vi "reward_behavior_timeout_12s_probes.vi"() -> ()   [LabVIEW 2019]
doc: "The myRIO Project template acquires acceleration data from the onboard accelerometer and displays the changes of acceleration values in a waveform chart."
uses:
  <vilib>/Analysis/Matrix/Datatypes/RealMatrix.ctl
  <vilib>/myRIO/Common/Instrument Driver Framework/myRIO v1.0/Encoder/typedefs/Encoder Signal Mode.ctl
  <vilib>/myRIO/Instrument Drivers/Onboard IO/Encoder/typedefs/Encoder Reference.ctl
  <vilib>/myRIO/Common/Instrument Driver Framework/Utilities/typedefs/myRIO Generic Hardware Reference.ctl
  <vilib>/myRIO/Common/Instrument Driver Framework/Utilities/typedefs/Hardware Version Enum.ctl
  <vilib>/myRIO/Common/Instrument Driver Framework/Utilities/typedefs/myRIO v1.0 Reference.ctl
  <vilib>/myRIO/Common/Instrument Driver Framework/Utilities/typedefs/Generic FPGA Reference.ctl
  <vilib>/myRIO/Common/Instrument Driver Framework/myRIO v1.0/Encoder/typedefs/Encoder Channels Enum.ctl
  <vilib>/myRIO/Common/Instrument Driver Framework/myRIO v1.0/Encoder/typedefs/Encoder Configuration v1.0.ctl
  <vilib>/userdefined/High Color/nirio_resource_hc.ctl
  <vilib>/myRIO/Instrument Drivers/Onboard IO/DIO/typedefs/DIO Reference.ctl
  <vilib>/myRIO/Common/Instrument Driver Framework/myRIO v1.0/DIO/typedefs/DIO Channels List.ctl
  <vilib>/myRIO/Common/Instrument Driver Framework/myRIO v1.0/DIO/typedefs/DIO Channels Enum.ctl
  <vilib>/myRIO/Common/Instrument Driver Framework/Utilities/vis/Is FPGA Ref Available.vi
  <vilib>/myRIO/Common/Instrument Driver Framework/myRIO v1.0/Encoder/vis/myRIO v1.1 Open Encoder.vi
  <vilib>/myRIO/Instrument Drivers/Onboard IO/Encoder/vis/Read.vi
  <vilib>/myRIO/Common/Instrument Driver Framework/myRIO v1.0/DIO/vis/myRIO v1.1 Open DIO.vi
  <vilib>/myRIO/Instrument Drivers/Onboard IO/DIO/vis/Write.vi
  <vilib>/myRIO/Instrument Drivers/Onboard IO/DIO/vis/Read.vi
  <vilib>/myRIO/Common/Instrument Driver Framework/Utilities/vis/Validate Channels.vi
  <vilib>/myRIO/Common/Instrument Driver Framework/myRIO v1.0/Encoder/vis/myRIO v1.0 Reserve Encoder.vi
  <vilib>/myRIO/Common/Instrument Driver Framework/myRIO v1.0/DIO/vis/myRIO v1.0 Reserve DIO.vi
  <vilib>/myRIO/Common/Instrument Driver Framework/myRIO v1.0/Encoder/vis/myRIO v1.0 Build MUX Configuration Encoder.vi
  <vilib>/myRIO/Common/Instrument Driver Framework/myRIO v1.0/Resource Manager/vis/myRIO v1.0 Reserve Channel List.vi
  <vilib>/myRIO/Common/Instrument Driver Framework/myRIO v1.0/DIO/vis/myRIO v1.0 Build MUX Configuration DIO.vi
  <vilib>/myRIO/Common/Instrument Driver Framework/myRIO v1.0/Resource Manager/vis/myRIO v1.0 Create Configuration List.vi
  <vilib>/myRIO/Common/Instrument Driver Framework/myRIO v1.0/Resource Manager/vis/myRIO v1.0 Reserve Channel.vi
  <vilib>/myRIO/Common/Instrument Driver Framework/myRIO v1.0/Resource Manager/vis/myRIO v1.0 Unreserve Channel.vi
  <vilib>/myRIO/Common/Instrument Driver Framework/myRIO v1.0/Resource Manager/vis/myRIO v1.0 Build Mutex Name.vi
  <vilib>/Utility/VariantDataType/GetNumericInfo.vi
  <vilib>/Utility/error.llb/Error Cluster From Error Code.vi
  <vilib>/myRIO/Common/Instrument Driver Framework/myRIO v1.0/myRIO v1.1 Open.vi
  <vilib>/myRIO/Common/Instrument Driver Framework/Utilities/vis/IO Manager.vi
  <vilib>/myRIO/Common/Instrument Driver Framework/Utilities/vis/Configuration Manager.vi
  <vilib>/myRIO/Common/Instrument Driver Framework/myRIO v1.0/Resource Manager/vis/myRIO v1.0 Configure IO.vi
  <vilib>/myRIO/Common/Instrument Driver Framework/myRIO v1.0/myRIO v1.0 Close.vi
  <vilib>/myRIO/Common/Instrument Driver Framework/myRIO v1.0/Encoder/vis/myRIO v1.0 Configure Encoder.vi
  <vilib>/myRIO/Common/Instrument Driver Framework/myRIO v1.0/Encoder/vis/myRIO v1.0 Read Encoder.vi
  <vilib>/myRIO/Common/Instrument Driver Framework/myRIO v1.0/DIO/vis/myRIO v1.0 Read DIO.vi
  <vilib>/myRIO/Common/Instrument Driver Framework/myRIO v1.0/DIO/vis/myRIO v1.0 Write DIO.vi
  <vilib>/myRIO/Express VI/Onboard IO/Encoder/Encoder Express VI.xnode
  <vilib>/myRIO/Instrument Drivers/Onboard IO/Encoder/vis/myRIO Encoder Open.xnode
  <vilib>/myRIO/Express VI/Onboard IO/DI/DI Express VI.xnode
  <vilib>/myRIO/Instrument Drivers/Onboard IO/DIO/vis/myRIO DIO Open.xnode
  <vilib>/myRIO/Express VI/Onboard IO/DO/DO Express VI.xnode
  <vilib>/myRIO/Instrument Drivers/Onboard IO/Encoder/Encoder.lvlib
  <vilib>/myRIO/Instrument Drivers/Onboard IO/DIO/DIO.lvlib
  <vilib>/Analysis/Matrix/NI_Matrix.lvlib
panel:
  out "Timings":dbl[](array[numeric])
  out "ISI":dbl
  out "ISI start time":dbl
  out "Time_out":bool=TRUE
  out "Time since lick":dbl
  out "Time of last lick":dbl
  out "Rewarded trials":dbl[](array[numeric])
  out "Rewards":u16
  out "Active Trial":bool
  out "Array temp2":T1
  out "Stimuli Loaded":bool
  out "Stim_ID":dbl[](array[numeric])
  out "Reward_mat":dbl[](array[numeric])
  out "Reward":bool=TRUE
  out "Frame clock":i32
  out "Licks":u32
  out "Lick":bool
  out "Time":dbl
  out "Stop":bool
  in  "Frames to collect":u32
  out "Overflow?":bool
  out "Counter Value":i32
  out "Velocity":dbl
  out "Velocity Plot":dbl[](graph)
  out "Velocity array":dbl[](array[numeric])
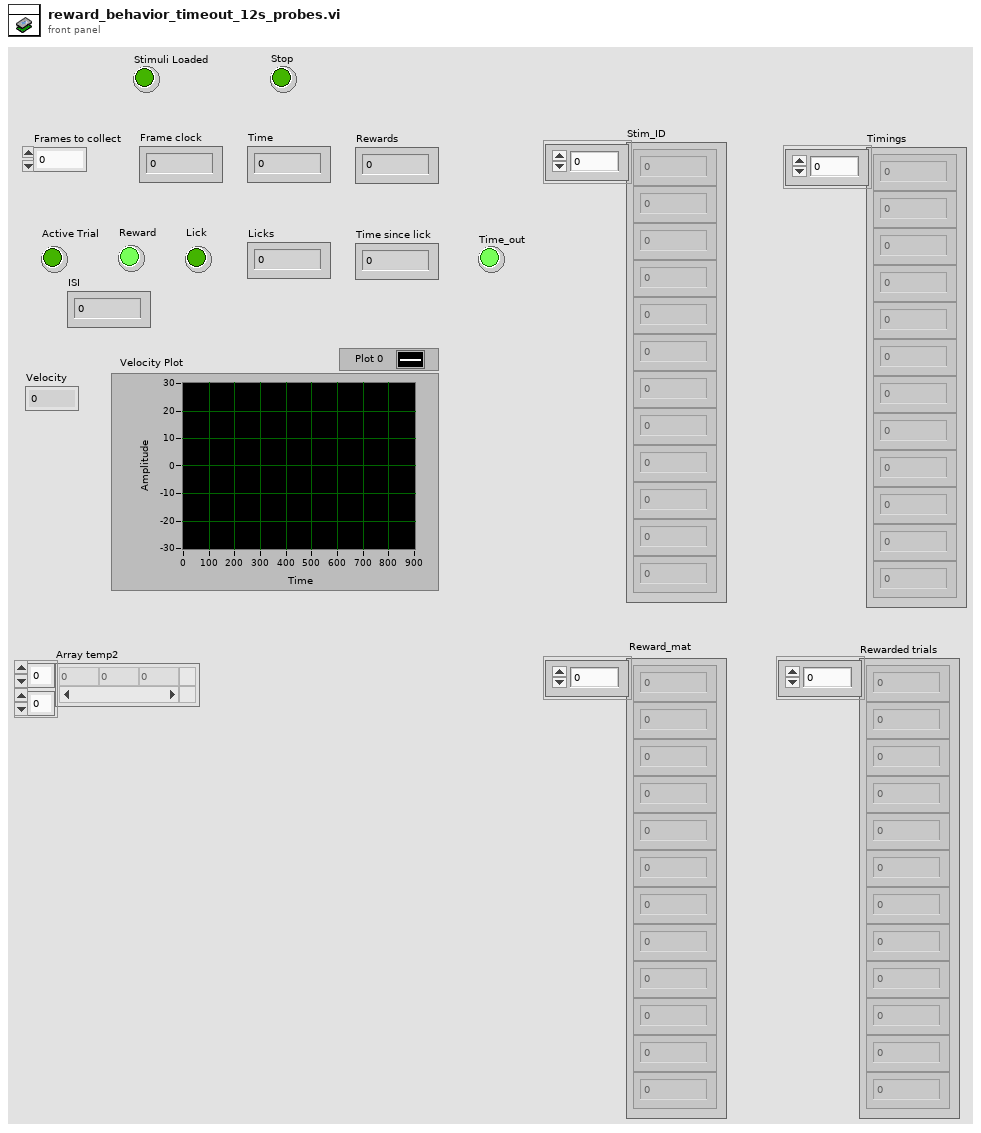
[diagram p1: front panel]
types:
  T1 = typedef "NI_Matrix.lvlib/RealMatrix.ctl" = dbl[][]
  T2 = typedef "Encoder.lvlib/Encoder Reference.ctl" = cluster{"myRIO Reference":T3, "Encoder Channels Enum":T7}
  T3 = typedef "myRIO Generic Hardware Reference.ctl" = cluster{"myRIO Model":T4, "myRIO Hardware Reference":T5}
  T4 = typedef "Hardware Version Enum.ctl" = enum16{"Unknown", "myRIO-1900", "myRIO-1950", "roboRIO", "NI ELVIS RIO CM", "ELVIS III"}
  T5 = typedef "myRIO v1.0 Reference.ctl" = cluster{"Generic FPGA Reference":T6, "Allow multiple opens":bool}
  T6 = typedef "Generic FPGA Reference.ctl" = refnum<k20>
  T7 = typedef "Encoder Channels Enum.ctl" = enum16{"Not Connected", "C/ENC0", "C/ENC1", "A/ENC", "A/ENC0", "A/ENC1", "A/ENC2", "A/ENC3", "A/ENC4", "A/ENC5", "A/ENC6", "A/ENC7", "A/ENC8", "A/ENC9", "B/ENC", "B/ENC0", "B/ENC1", "B/ENC2", "B/ENC3", "B/ENC4", "B/ENC5", "B/ENC6", "B/ENC7", "B/ENC8", "B/ENC9", "DIO/ENC0", "DIO/ENC1", "DIO/ENC2", "DIO/ENC3", "DIO/ENC4"}
  T8 = typedef "Encoder Signal Mode.ctl" = enum16{"Quadrature phase signal", "Step and direction signal"}
  T9 = typedef "nirio_resource_hc.ctl" = tag
  T10 = typedef "DIO.lvlib/DIO Reference.ctl" = cluster{"myRIO Reference":T3, "DIO Channels List":T11}
  T11 = typedef "DIO Channels List.ctl" = T12[]
  T12 = typedef "DIO Channels Enum.ctl" = enum16{"Not Connected", "C/DIO0", "C/DIO1", "C/DIO2", "C/DIO3", "C/DIO4", "C/DIO5", "C/DIO6", "C/DIO7", "A/DIO0", "A/DIO1", "A/DIO2", "A/DIO3", "A/DIO4", "A/DIO5", "A/DIO6", "A/DIO7", "A/DIO8", "A/DIO9", "A/DIO10", "A/DIO11", "A/DIO12", "A/DIO13", "A/DIO14", "A/DIO15", "A/DIO16", "A/DIO17", "A/DIO18", "A/DIO19", "B/DIO0", "B/DIO1", "B/DIO2", "B/DIO3", "B/DIO4", "B/DIO5", "B/DIO6", "B/DIO7", "B/DIO8", "B/DIO9", "B/DIO10", "B/DIO11", "B/DIO12", "B/DIO13", "B/DIO14", "B/DIO15", "B/DIO16", "B/DIO17", "B/DIO18", "B/DIO19", "LED0", "LED1", "LED2", "LED3", "Button0", "DIO/DIO0", "DIO/DIO1", "DIO/DIO2", "DIO/DIO3", "DIO/DIO4", "DIO/DIO5", "DIO/DIO6", "DIO/DIO7", "DIO/DIO8", "DIO/DIO9", "SPI/CS0", "SPI/CS1", "SPI/CS2", "SPI/CS3", "LED RADIO (Green)", "LED RADIO (Red)", "LED COMM (Green)", "LED COMM (Red)", "LED MODE (Green)", "LED MODE (Red)"}
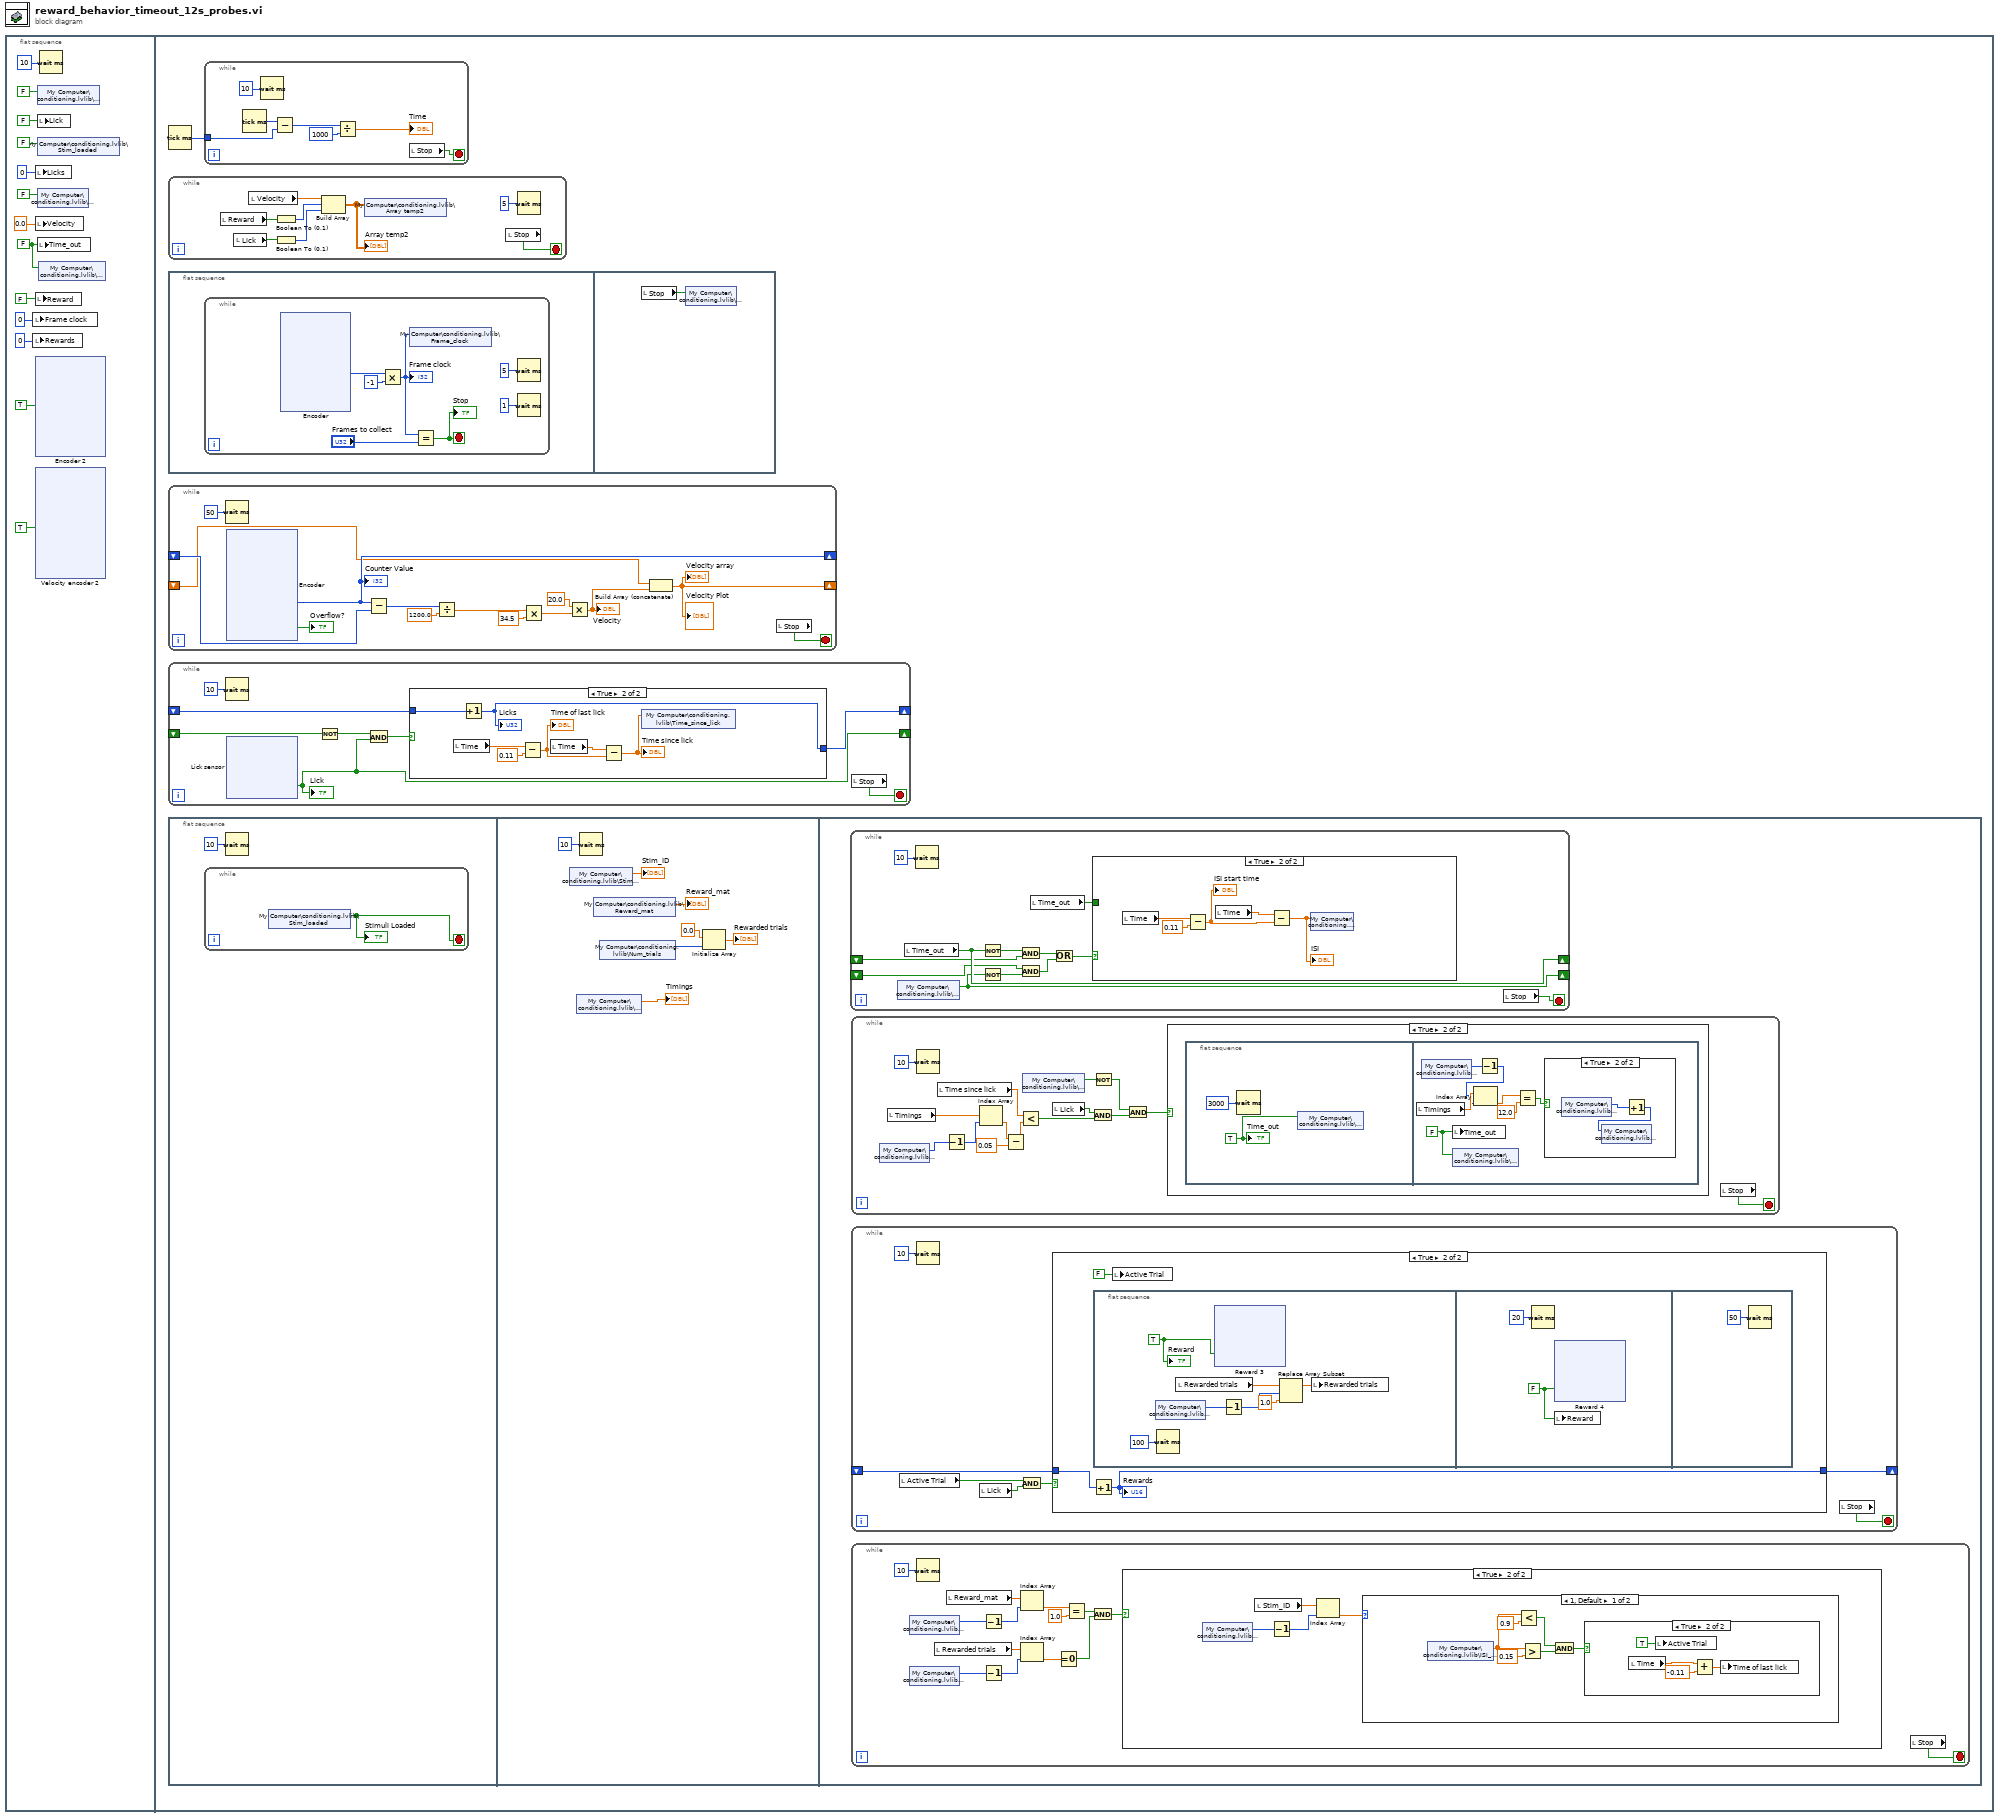
[diagram p0: block diagram]
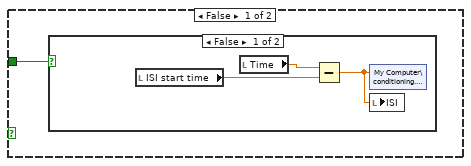
[diagram p4: hidden frame]
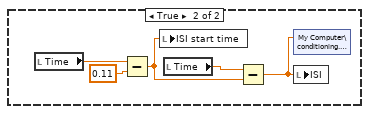
[diagram p5: hidden frame]
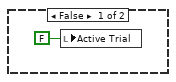
[diagram p6: hidden frame]
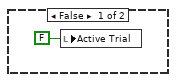
[diagram p7: hidden frame]
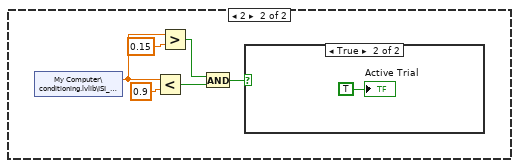
[diagram p8: hidden frame]
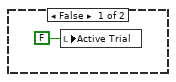
[diagram p9: hidden frame]
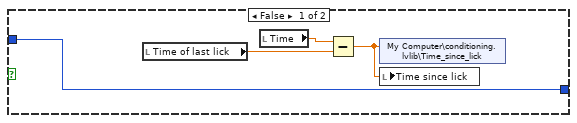
[diagram p11: hidden frame]
diagram:
  n1 = flat-sequence {
    frame #0 {
      w1 = FALSE ("Time_out")
      n2 = local write "Frame clock"(u32 0 ("Frames")) -> ()
      n3 = local write "Rewards"(u16 0 ("Rewards")) -> ()
      n4 = local write "Licks"(u32 0 ("Licks")) -> ()
      n5 = local write "Velocity"(0.0 ("Velocity")) -> ()
      n6 = local write "Reward"(FALSE ("Give reward")) -> ()
      n7 = xnode "Encoder 2"("Reset Counter"=TRUE) -> ()  [unwired: 1 in, 4 out]
      n8 = xnode "Velocity encoder 2"("Reset Counter"=TRUE) -> ()  [unwired: 1 in, 4 out]
      n9 = shared-variable "My Computer\\conditioning.lvlib\\Display"(FALSE ("Display")) -> ()  [unwired: 1 in, 1 out]
      n10 = local write "Lick"(FALSE ("Lick")) -> ()
      n11 = shared-variable "My Computer\\conditioning.lvlib\\Stim_loaded"(FALSE ("Stim_loaded")) -> ()  [unwired: 1 in, 1 out]
      n12 = shared-variable "My Computer\\conditioning.lvlib\\Stop"(FALSE ("Stop")) -> ()  [unwired: 1 in, 1 out]
      n13 = local write "Time_out"(w1) -> ()
      n14 = shared-variable "My Computer\\conditioning.lvlib\\Timeout"(w1) -> ()  [unwired: 1 in, 1 out]
      n15 = Wait (ms)(milliseconds to wait=u32 10) -> ()  [unwired: 1 out]
    }
    frame #1 {
      n16 = Tick Count (ms)() -> (millisecond timer value=w106:u32)
      n17 = while {
        stop <- w108 stop-if-true
        n18 = local read "Reward"() -> (w113:bool)
        n19 = local read "Lick"() -> (w114:bool)
        n20 = local read "Velocity"() -> (w112:dbl)
        n21 = Boolean To (0,1)(Boolean=w113) -> (0, 1=w111:i16)
        n22 = Boolean To (0,1)(Boolean=w114) -> (0, 1=w110:i16)
        n23 = Build Array(w112, w111, w110) -> (w107:T1)
        "Array temp2" <- w107
        n24 = shared-variable "My Computer\\conditioning.lvlib\\Array temp2"(w107) -> ()  [unwired: 1 in, 1 out]
        n25 = local read "Stop"() -> (w108:bool)
        n26 = Wait (ms)(milliseconds to wait=u32 5) -> ()  [unwired: 1 out]
      }
      n27 = flat-sequence {
        frame #0 {
          n28 = while {
            stop <- w306 stop-if-true
            n29 = xnode "Encoder"() -> ("Counter Value"=w310:i32)  [unwired: 2 in, 3 out]
            n30 = Multiply(x=w310, y=-1) -> (x*y=w305:i32)
            "Frame clock" <- w305
            n31 = shared-variable "My Computer\\conditioning.lvlib\\Frame_clock"(w305) -> ()  [unwired: 1 in, 1 out]
            n32 = Equal?(x=w305, y="Frames to collect") -> (x = y?=w306:bool)
            "Stop" <- w306
            n33 = Wait (ms)(milliseconds to wait=u32 5) -> ()  [unwired: 1 out]
            n34 = Wait (ms)(milliseconds to wait=u32 1) -> ()  [unwired: 1 out]
          }
        }
        frame #1 {
          n35 = local read "Stop"() -> (w358:bool)
          n36 = shared-variable "My Computer\\conditioning.lvlib\\Stop"(w358) -> ()  [unwired: 1 in, 1 out]
        }
      }
      n37 = while {
        shift-right: [w423] -> _
        shift-left: _ -> [w424]
        shift-right: [w415] -> _
        shift-left: _ -> [w414]
        stop <- w413 stop-if-true
        n38 = Wait (ms)(milliseconds to wait=u32 50) -> ()  [unwired: 1 out]
        n39 = xnode "Encoder"() -> ("Counter Value"=w423:i32, "Overflow?"=→"Overflow?":bool)  [unwired: 2 in, 2 out]
        "Counter Value" <- w423
        n40 = Subtract(x=w423, y=w424) -> (x-y=w416:i32)
        n41 = Divide(x=w416, y=1200.0 ("600")) -> (x/y=w421:dbl)
        n42 = Multiply(x=w421, y=34.5) -> (x*y=w419:dbl)
        n43 = Multiply(x=20.0, y=w419) -> (x*y=w417:dbl)
        "Velocity" <- w417
        n44 = Build Array (concatenate)(w414, w417) -> (w415:dbl[])
        "Velocity Plot" <- w415
        "Velocity array" <- w415
        n45 = local read "Stop"() -> (w413:bool)
      }
      n46 = while {
        shift-right: [w365] -> _
        shift-left: _ -> [w364]
        shift-right: [w359] -> _
        shift-left: _ -> [w362]
        stop <- w363 stop-if-true
        n47 = Wait (ms)(milliseconds to wait=u32 10) -> ()  [unwired: 1 out]
        n48 = xnode "Lick sensor"() -> ("C/DIO1 (DIO1)"=w359:bool)  [unwired: 1 in, 1 out]
        "Lick" <- w359
        n49 = Not(x=w362) -> (.not. x?=w361:bool)
        n50 = And(x=w361, y=w359) -> (x .and. y?=w360:bool)
        n51 = case shown="True" w360 {
          tunnel: [w370 w377] -> w365
          tunnel: w364 -> [w370 w376]
          frame False {
            n52 = local read "Time of last lick"() -> (w368:dbl)
            n53 = local read "Time"() -> (w369:dbl)
            n54 = Subtract(x=w369, y=w368) -> (x-y=w367:dbl)
            n55 = shared-variable "My Computer\\conditioning.lvlib\\Time_since_lick"(w367) -> ()  [unwired: 1 in, 1 out]
            n56 = local write "Time since lick"(w367) -> ()
          }
          frame True {
            n57 = local read "Time"() -> (w373:dbl)
            n58 = Increment(x=w376) -> (x+1=w377:u32)
            "Licks" <- w377
            n59 = Subtract(x=w373, y=0.11) -> (x-y=w371:dbl)
            "Time of last lick" <- w371
            n60 = local read "Time"() -> (w375:dbl)
            n61 = Subtract(x=w375, y=w371) -> (x-y=w374:dbl)
            "Time since lick" <- w374
            n62 = shared-variable "My Computer\\conditioning.lvlib\\Time_since_lick"(w374) -> ()  [unwired: 1 in, 1 out]
          }
        }
        n63 = local read "Stop"() -> (w363:bool)
      }
      n64 = flat-sequence {
        frame #0 {
          n65 = while {
            stop <- w116 stop-if-true
            n66 = shared-variable "My Computer\\conditioning.lvlib\\Stim_loaded"() -> (w116:bool)  [unwired: 1 in, 1 out]
            "Stimuli Loaded" <- w116
          }
          n67 = Wait (ms)(milliseconds to wait=u32 10) -> ()  [unwired: 1 out]
        }
        frame #1 {
          n68 = shared-variable "My Computer\\conditioning.lvlib\\Stim_ID"() -> (→"Stim_ID":dbl[])  [unwired: 1 in, 1 out]
          n69 = shared-variable "My Computer\\conditioning.lvlib\\Timings"() -> (→"Timings":dbl[])  [unwired: 1 in, 1 out]
          n70 = Wait (ms)(milliseconds to wait=u32 10) -> ()  [unwired: 1 out]
          n71 = shared-variable "My Computer\\conditioning.lvlib\\Reward_mat"() -> (→"Reward_mat":dbl[])  [unwired: 1 in, 1 out]
          n72 = shared-variable "My Computer\\conditioning.lvlib\\Num_trials"() -> (w120:u32)  [unwired: 1 in, 1 out]
          n73 = Initialize Array(0.0 ("element"), w120) -> (→"Rewarded trials":dbl[])
        }
        frame #2 {
          n74 = while {
            shift-right: [w160] -> _
            shift-left: _ -> [w158]
            shift-right: [w156] -> _
            shift-left: _ -> [w155]
            stop <- w161 stop-if-true
            n75 = shared-variable "My Computer\\conditioning.lvlib\\Display"() -> (w156:bool)  [unwired: 1 in, 1 out]
            n76 = local read "Time_out"() -> (w160:bool)
            n77 = Wait (ms)(milliseconds to wait=u32 10) -> ()  [unwired: 1 out]
            n78 = Not(x=w160) -> (.not. x?=w159:bool)
            n79 = Not(x=w156) -> (.not. x?=w154:bool)
            n80 = And(x=w159, y=w158) -> (x .and. y?=w153:bool)
            n81 = And(x=w155, y=w154) -> (x .and. y?=w152:bool)
            n82 = local read "Time_out"() -> (w157:bool)
            n83 = Or(x=w153, y=w152) -> (x .or. y?=w151:bool)
            n84 = case shown="True" w151 {
              tunnel: w157 -> [w162 _]
              frame False {
                n85 = case shown="False" w162 {
                  frame False {
                    n86 = local read "ISI start time"() -> (w165:dbl)
                    n87 = local read "Time"() -> (w164:dbl)
                    n88 = Subtract(x=w164, y=w165) -> (x-y=w163:dbl)
                    n89 = shared-variable "My Computer\\conditioning.lvlib\\ISI"(w163) -> ()  [unwired: 1 in, 1 out]
                    n90 = local write "ISI"(w163) -> ()
                  }
                  frame True {
                    n91 = local read "Time"() -> (w170:dbl)
                    n92 = Subtract(x=w170, y=0.11) -> (x-y=w167:dbl)
                    n93 = local write "ISI start time"(w167) -> ()
                    n94 = local read "Time"() -> (w168:dbl)
                    n95 = Subtract(x=w168, y=w167) -> (x-y=w166:dbl)
                    n96 = shared-variable "My Computer\\conditioning.lvlib\\ISI"(w166) -> ()  [unwired: 1 in, 1 out]
                    n97 = local write "ISI"(w166) -> ()
                  }
                }
              }
              frame True {
                n98 = local read "Time"() -> (w175:dbl)
                n99 = Subtract(x=w175, y=0.11) -> (x-y=w172:dbl)
                "ISI start time" <- w172
                n100 = local read "Time"() -> (w173:dbl)
                n101 = Subtract(x=w173, y=w172) -> (x-y=w171:dbl)
                "ISI" <- w171
                n102 = shared-variable "My Computer\\conditioning.lvlib\\ISI"(w171) -> ()  [unwired: 1 in, 1 out]
              }
            }
            n103 = local read "Stop"() -> (w161:bool)
          }
          n104 = while {
            stop <- w138 stop-if-true
            n105 = shared-variable "My Computer\\conditioning.lvlib\\Trial"() -> (w128:u32)  [unwired: 1 in, 1 out]
            n106 = local read "Timings"() -> (w129:dbl[])
            n107 = Wait (ms)(milliseconds to wait=u32 10) -> ()  [unwired: 1 out]
            n108 = local read "Time since lick"() -> (w137:dbl)
            n109 = Decrement(x=w128) -> (x-1=w127:u32)
            n110 = Index Array(array=w129, index=w127) -> (element=w125:dbl)
            n111 = Subtract(x=w125, y=0.05) -> (x-y=w124:dbl)
            n112 = Less?(x=w137, y=w124) -> (x < y?=w136:bool)
            n113 = shared-variable "My Computer\\conditioning.lvlib\\Display"() -> (w133:bool)  [unwired: 1 in, 1 out]
            n114 = local read "Lick"() -> (w135:bool)
            n115 = Not(x=w133) -> (.not. x?=w132:bool)
            n116 = And(x=w135, y=w136) -> (x .and. y?=w131:bool)
            n117 = And(x=w132, y=w131) -> (x .and. y?=w130:bool)
            n118 = case shown="True" w130 {
              frame False {
              }
              frame True {
                n119 = flat-sequence {
                  frame #0 {
                    w140 = TRUE
                    n120 = Wait (ms)(milliseconds to wait=u32 3000) -> ()  [unwired: 1 out]
                    n121 = shared-variable "My Computer\\conditioning.lvlib\\Timeout"(w140) -> ()  [unwired: 1 in, 1 out]
                    "Time_out" <- w140
                  }
                  frame #1 {
                    w147 = FALSE ("Timeout")
                    n122 = local read "Timings"() -> (w146:dbl[])
                    n123 = shared-variable "My Computer\\conditioning.lvlib\\Trial"() -> (w142:u32)  [unwired: 1 in, 1 out]
                    n124 = local write "Time_out"(w147) -> ()
                    n125 = shared-variable "My Computer\\conditioning.lvlib\\Timeout"(w147) -> ()  [unwired: 1 in, 1 out]
                    n126 = Decrement(x=w142) -> (x-1=w141:u32)
                    n127 = Index Array(array=w146, index=w141) -> (element=w144:dbl)
                    n128 = Equal?(x=w144, y=12.0) -> (x = y?=w145:bool)
                    n129 = case shown="True" w145 {
                      frame False {
                      }
                      frame True {
                        n130 = shared-variable "My Computer\\conditioning.lvlib\\Trial"() -> (w149:u32)  [unwired: 1 in, 1 out]
                        n131 = Increment(x=w149) -> (x+1=w148:u32)
                        n132 = shared-variable "My Computer\\conditioning.lvlib\\Trial"(w148) -> ()  [unwired: 1 in, 1 out]
                      }
                    }
                  }
                }
              }
            }
            n133 = local read "Stop"() -> (w138:bool)
          }
          n134 = while {
            shift-right: [w217] -> _
            shift-left: _ -> [w216]
            stop <- w220 stop-if-true
            n135 = local read "Active Trial"() -> (w214:bool)
            n136 = Wait (ms)(milliseconds to wait=u32 10) -> ()  [unwired: 1 out]
            n137 = local read "Lick"() -> (w215:bool)
            n138 = And(x=w214, y=w215) -> (x .and. y?=w218:bool)
            n139 = case shown="True" w218 {
              tunnel: [w221 w224] -> w217
              tunnel: w216 -> [w221 w223]
              frame False {
              }
              frame True {
                n140 = Increment(x=w223) -> (x+1=w224:u16)
                "Rewards" <- w224
                n141 = flat-sequence {
                  frame #0 {
                    w230 = TRUE ("C/DIO0 (DIO0)")
                    n142 = shared-variable "My Computer\\conditioning.lvlib\\Trial"() -> (w229:u32)  [unwired: 1 in, 1 out]
                    n143 = Wait (ms)(milliseconds to wait=u32 100) -> ()  [unwired: 1 out]
                    n144 = local read "Rewarded trials"() -> (w227:dbl[])
                    n145 = xnode "Reward 3"("C/DIO0 (DIO0)"=w230) -> ()  [unwired: 1 in, 1 out]
                    n146 = Decrement(x=w229) -> (x-1=w228:u32)
                    n147 = Replace Array Subset(array=w227, new element=1.0 ("new element/subarray"), index=w228) -> (w225:dbl[])
                    n148 = local write "Rewarded trials"(w225) -> ()
                    "Reward" <- w230
                  }
                  frame #1 {
                    w268 = FALSE ("C/DIO0 (DIO0)")
                    n149 = Wait (ms)(milliseconds to wait=u32 20) -> ()  [unwired: 1 out]
                    n150 = xnode "Reward 4"("C/DIO0 (DIO0)"=w268) -> ()  [unwired: 1 in, 1 out]
                    n151 = local write "Reward"(w268) -> ()
                  }
                  frame #2 {
                    n152 = Wait (ms)(milliseconds to wait=u32 50) -> ()  [unwired: 1 out]
                  }
                }
                n153 = local write "Active Trial"(FALSE ("Active Trial")) -> ()
              }
            }
            n154 = local read "Stop"() -> (w220:bool)
          }
          n155 = while {
            stop <- w189 stop-if-true
            n156 = shared-variable "My Computer\\conditioning.lvlib\\Trial"() -> (w185:u32)  [unwired: 1 in, 1 out]
            n157 = shared-variable "My Computer\\conditioning.lvlib\\Trial"() -> (w181:u32)  [unwired: 1 in, 1 out]
            n158 = Wait (ms)(milliseconds to wait=u32 10) -> ()  [unwired: 1 out]
            n159 = local read "Rewarded trials"() -> (w182:dbl[])
            n160 = local read "Reward_mat"() -> (w184:dbl[])
            n161 = Decrement(x=w185) -> (x-1=w186:u32)
            n162 = Decrement(x=w181) -> (x-1=w180:u32)
            n163 = Index Array(array=w184, index=w186) -> (element=w187:dbl)
            n164 = Index Array(array=w182, index=w180) -> (element=w179:dbl)
            n165 = Equal To 0?(x=w179) -> (x = 0?=w178:bool)
            n166 = Equal?(x=w187, y=1.0) -> (x = y?=w177:bool)
            n167 = And(x=w177, y=w178) -> (x .and. y?=w176:bool)
            n168 = case shown="True" w176 {
              frame False {
                n169 = local write "Active Trial"(FALSE ("Active_trial")) -> ()
              }
              frame True {
                n170 = shared-variable "My Computer\\conditioning.lvlib\\Trial"() -> (w192:u32)  [unwired: 1 in, 1 out]
                n171 = local read "Stim_ID"() -> (w194:dbl[])
                n172 = Decrement(x=w192) -> (x-1=w193:u32)
                n173 = Index Array(array=w194, index=w193) -> (element=w191:dbl)
                n174 = case shown="1, Default" w191 {
                  frame 1, Default {
                    n175 = shared-variable "My Computer\\conditioning.lvlib\\ISI_Time"() -> (w199:dbl)  [unwired: 1 in, 1 out]
                    n176 = Less?(x=w199, y=0.9) -> (x < y?=w197:bool)
                    n177 = Greater?(x=w199, y=0.15) -> (0:w196:bool)
                    n178 = And(x=w197, y=w196) -> (x .and. y?=w195:bool)
                    n179 = case shown="True" w195 {
                      frame False {
                        n180 = local write "Active Trial"(FALSE ("Active Trial")) -> ()
                      }
                      frame True {
                        n181 = local read "Time"() -> (w204:dbl)
                        n182 = local write "Active Trial"(TRUE ("Active Trial")) -> ()
                        n183 = Add(x=w204, y=-0.11) -> (x+y=w202:dbl)
                        n184 = local write "Time of last lick"(w202) -> ()
                      }
                    }
                  }
                  frame 2 {
                    n185 = shared-variable "My Computer\\conditioning.lvlib\\ISI_Time"() -> (w210:dbl)  [unwired: 1 in, 1 out]
                    n186 = Less?(x=w210, y=0.9) -> (x < y?=w207:bool)
                    n187 = Greater?(x=w210, y=0.15) -> (0:w208:bool)
                    n188 = And(x=w208, y=w207) -> (x .and. y?=w206:bool)
                    n189 = case shown="True" w206 {
                      frame False {
                        n190 = local write "Active Trial"(FALSE ("Active Trial")) -> ()
                      }
                      frame True {
                        "Active Trial" <- TRUE ("Active Trial")
                      }
                    }
                  }
                }
              }
            }
            n191 = local read "Stop"() -> (w189:bool)
          }
        }
      }
      n192 = while {
        tunnel: w106 -> [w478]
        stop <- w476 stop-if-true
        n193 = Tick Count (ms)() -> (millisecond timer value=w479:u32)
        n194 = Wait (ms)(milliseconds to wait=u32 10) -> ()  [unwired: 1 out]
        n195 = Subtract(x=w479, y=w478) -> (x-y=w475:u32)
        n196 = Divide(x=w475, y=u32 1000) -> (x/y=→"Time":dbl)
        n197 = local read "Stop"() -> (w476:bool)
      }
    }
  }
